vi "Square Wave 2.vi"(0 "samples":i32=128, 2 "amplitude":dbl=1.0 format="%.2f", 4 "duty (ticks)":u32=50, 5 "phase ticks":dbl format="%.2f") -> (6 "Square Wave":dbl[](array[numeric]) format="%.2f", 8 "error":i32)   [LabVIEW 2010]
doc: "This VI generates an array containing a square wave. If Square Wave is represented by the sequence Y, the VI generates the pattern according to the following formula:\n\n y[i] = amp * square(phase[i]), for i = 0, 1, 2, ..., n-1,\n\n where \n amp = amplitude\n n = number of samples\n \n square[p] = \n 1.0 if 0 <= pmod < (0.01*duty) * 360.0\n -1.0 if (0.01*duty) * 360.0 <= pmod < 360.0\n where pmod = p modulo 360.0\n duty = duty cycle in percent\n\n phase[i] = initial_phase + f*360.0*i\n where \n f = normalized frequency (cycles/sample )\n initial_phase = phase in, if reset phase is true\n = last output phase, if reset phase is false\n\nThis VI is reentrant so that it can be used to simulate a continuous acquisition from a square wave function generator. If the input control reset phase is false, subsequent calls to this VI will produce the output Square Wave array containing the NEXT n samples of a square wave.\n\n phase out is set to phase[n], and this reentrant VI will use this value as its new phase in if reset phase is false the next time the VI is executed."
uses:
  <vilib>/Analysis/NI_AALBase.lvlib
panel:
  # "Square Wave"
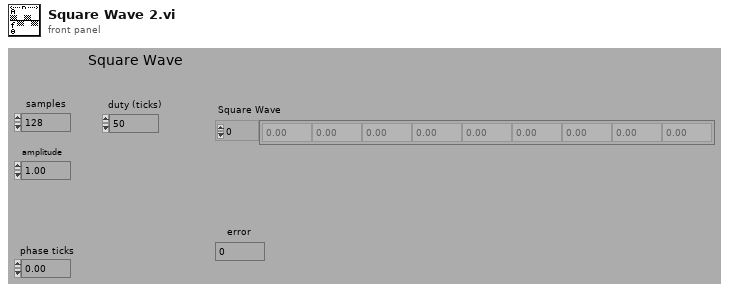
[diagram p1: front panel]
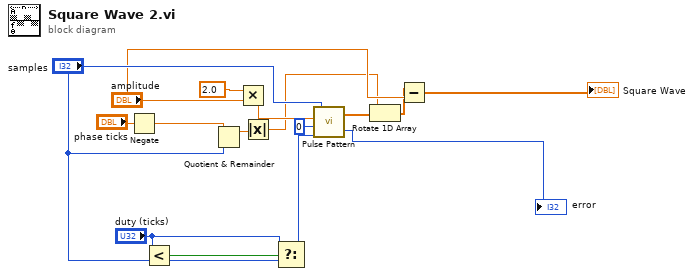
[diagram p0: block diagram]
diagram:
  n1 = Negate(x="phase ticks") -> (-x=w6:dbl)
  n2 = Less?(x="duty (ticks)", y="samples") -> (x < y?=w12:bool)
  n3 = Quotient & Remainder(x=w6, y="samples") -> (x-y*floor(x/y)=w5:dbl)  [unwired: 1 out]
  n4 = Multiply(x=2.0, y="amplitude") -> (x*y=w14:dbl)
  n5 = Absolute Value(x=w5) -> (abs(x)=w3:dbl)
  n6 = Select(t="duty (ticks)", s=w12, f="samples") -> (s? t:f=w10:u32)
  n7 = call <vilib>:"Pulse Pattern.vi"("width"=w10, "delay"=0, "amplitude"=w14, "samples"="samples") -> ("error"=→"error":i32, "Pulse Pattern"=w2:dbl[])
  n8 = Rotate 1D Array(1:w2, 2:w3) -> (0:w1:dbl[])
  n9 = Subtract(x=w1, y="amplitude") -> (x-y=→"Square Wave":dbl[])
